vi "Temperature.vi"(11 "Output All":string) -> (3 "Temperature (C)":string)   [LabVIEW 2015]
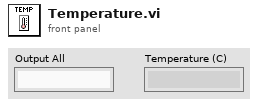
[diagram p1: front panel]
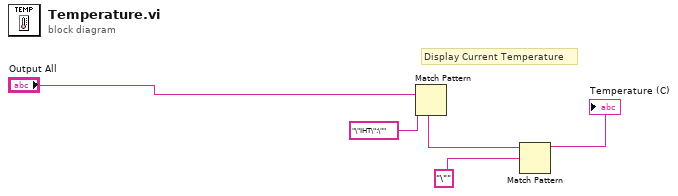
[diagram p0: block diagram]
diagram:
  # "Display Current Temperature"
  n1 = Match Pattern(string="Output All", regular expression="\"IHT\":\"") -> (after substring=w2:string)  [unwired: 1 in, 3 out]
  n2 = Match Pattern(string=w2, regular expression="\"") -> (before substring=→"Temperature (C)":string)  [unwired: 1 in, 3 out]
